vi "TCP_ReadACK.vi"(8 "error in (no error)":errorcluster, 11 "TCP Network Connection in":refnum<k5>) -> (0 "error out":errorcluster, 2 "Driver response":bool, 3 "TCP Network Connection out":refnum<k5>)   [LabVIEW 2019]
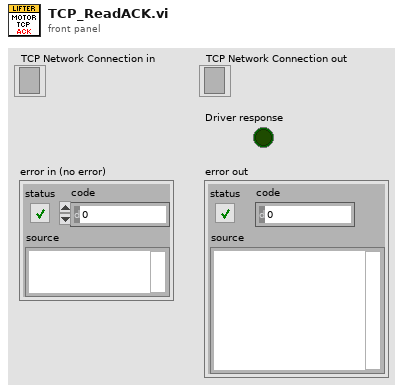
[diagram p1: front panel]
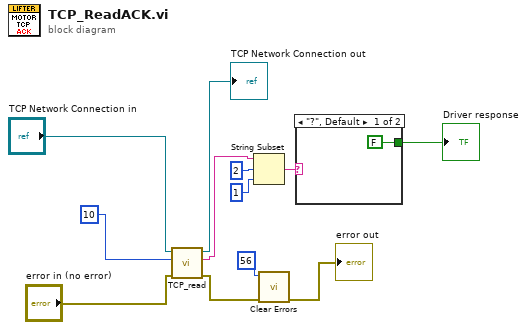
[diagram p0: block diagram]
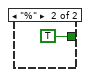
[diagram p2: hidden frame]
diagram:
  n1 = call "TCP_read.vi"("error in (no error)"="error in (no error)", "bytes to read"=10, "TCP Network Connection in"="TCP Network Connection in") -> ("error out"=w5:errorcluster, "DataOut"=w1:string, "TCP Network Connection out"=→"TCP Network Connection out":refnum<k5>)  [unwired: 6 in]
  n2 = String Subset(string=w1, offset (0)=2, length (rest)=1 ("length (rest)")) -> (substring=w9:string)
  n3 = call <vilib>:"Clear Errors.vi"("error in (no error)"=w5, "specific error code to clear (0: all)"=56) -> ("error out"=→"error out":errorcluster)  [unwired: 4 in, 1 out]
  n4 = case shown="\"?\", Default" w9 {
    tunnel: [FALSE ("Command Executed 2") TRUE ("Command Executed 2")] -> w12
    frame "?", Default {
    }
    frame "%" {
    }
  }
  "Driver response" <- w12
